vi "Fan_unit.vi"() -> (1 "Temperature (ADC value)":u8, 9 "Fan speed (DAC Value)":u8)   [LabVIEW 2024]
uses:
  Global 1.vi
panel:
  out "Heating (const)":dbl
  out "Fan speed (RPM)":dbl
  out "Total Cooling":dbl
  out "Temperature (deg C)":dbl
  in  "5V power":bool
  in  "9V power":bool
  # "FAN UNIT SIMULATOR"
  # "ON"
  # "OFF"
  # "9V power for fan\n5V power for heater and temperature sensor"
  # "K8055 SIGNALS\n(IN GLOBAL VARIABLE)"
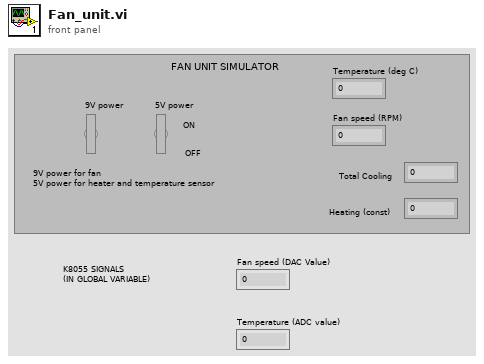
[diagram p1: front panel]
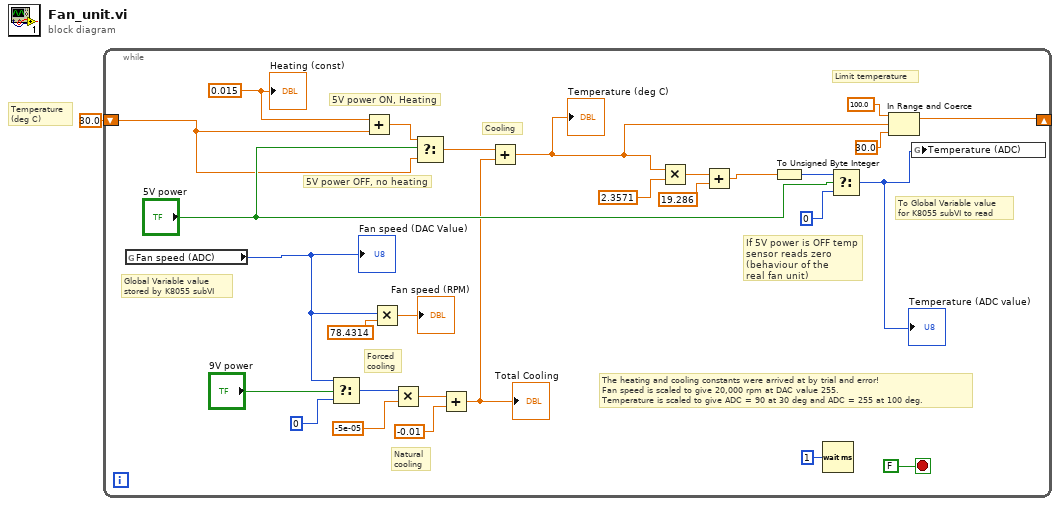
[diagram p0: block diagram]
diagram:
  # "Temperature\n(deg C)"
  n1 = while {
    shift-right: [w22] -> _
    shift-left: 30.0 -> [w4]
    stop <- FALSE stop-if-true
    w5 = 0.015 ("y")
    # "Limit temperature"
    # "5V power OFF, no heating"
    # "The heating and cooling constants were arrived at by trial and error!\nFan speed is scaled to give 20,000 rpm at DAC value 255.\nTemperature is scaled to give ADC = 90 at 30 deg and ADC = 255 at 100 deg."
    # "If 5V power is OFF temp\nsensor reads zero\n(behaviour of the\nreal fan unit)"
    # "Natural\ncooling"
    # "Forced\ncooling"
    # "Cooling"
    # "5V power ON, Heating"
    # "To Global Variable value\nfor K8055 subVI to read"
    # "Global Variable value\nstored by K8055 subVI"
    n2 = global read "Global 1.vi" "Fan speed (ADC)"() -> (w3:u8)
    "Fan speed (DAC Value)" <- w3
    n3 = Select(t=w3, s="9V power", f=u8 0) -> (s? t:f=w16:u8)
    n4 = Add(x=w5, y=w4) -> (x+y=w19:dbl)
    n5 = Multiply(x=w3, y=78.4314) -> (x*y=→"Fan speed (RPM)":dbl)
    n6 = Multiply(x=w16, y=-5e-05) -> (x*y=w15:dbl)
    n7 = Select(t=w19, s="5V power", f=w4) -> (s? t:f=w13:dbl)
    n8 = Add(x=w15, y=-0.01) -> (x+y=w12:dbl)
    "Total Cooling" <- w12
    n9 = Add(x=w13, y=w12) -> (x+y=w11:dbl)
    "Temperature (deg C)" <- w11
    n10 = Multiply(x=w11, y=2.3571) -> (x*y=w10:dbl)
    n11 = Add(x=w10, y=19.286) -> (x+y=w8:dbl)
    n12 = To Unsigned Byte Integer(number=w8) -> (unsigned 8bit integer=w21:u8)
    n13 = Wait (ms)(milliseconds to wait=u32 1) -> ()  [unwired: 1 out]
    n14 = Select(t=w21, s="5V power", f=u8 0) -> (s? t:f=w2:u8)
    "Temperature (ADC value)" <- w2
    n15 = In Range and Coerce(upper limit=100.0, x=w11, lower limit=30.0) -> (coerced(x)=w22:dbl)  [unwired: 1 out]
    n16 = global write "Global 1.vi" "Temperature (ADC)"(w2) -> ()
    "Heating (const)" <- w5
  }
